vi "Apply Body Text.vi"(6 "Layer name":string, 8 "error in (no error)":errorcluster, 9 "Body test":T2 {"Body Text Spec"."Alignment" items=["left", "center", "right"]}, 10 "Path & Icon":T5, 11 "Icon in":refnum<class "Icon.lvclass">) -> (0 "error out":errorcluster, 2 "Data":T1 {"Opacity" scale=0.0..100.0}, 3 "Icon out":refnum<class "Icon.lvclass">)   [LabVIEW 2021, in "Icon.lvclass"]
doc: "Updates the Text of the Text Layer."
uses:
  <vilib>/LabVIEW Icon API/lv_icon/Classes/Icon/Icon.lvclass
  <vilib>/LabVIEW Icon API/lv_icon/Controls/Graphic.ctl
  <vilib>/LabVIEW Icon API/lv_icon/Controls/BodyText.ctl
  <vilib>/LabVIEW Icon API/lv_icon/Controls/Font.ctl
  <vilib>/LabVIEW Icon API/lv_icon/Controls/Alignment.ctl
  <vilib>/LabVIEW Icon API/lv_icon/Controls/Layer.ctl
  <vilib>/LabVIEW Icon API/lv_icon/Classes/Icon Framework/Icon Framework.lvclass
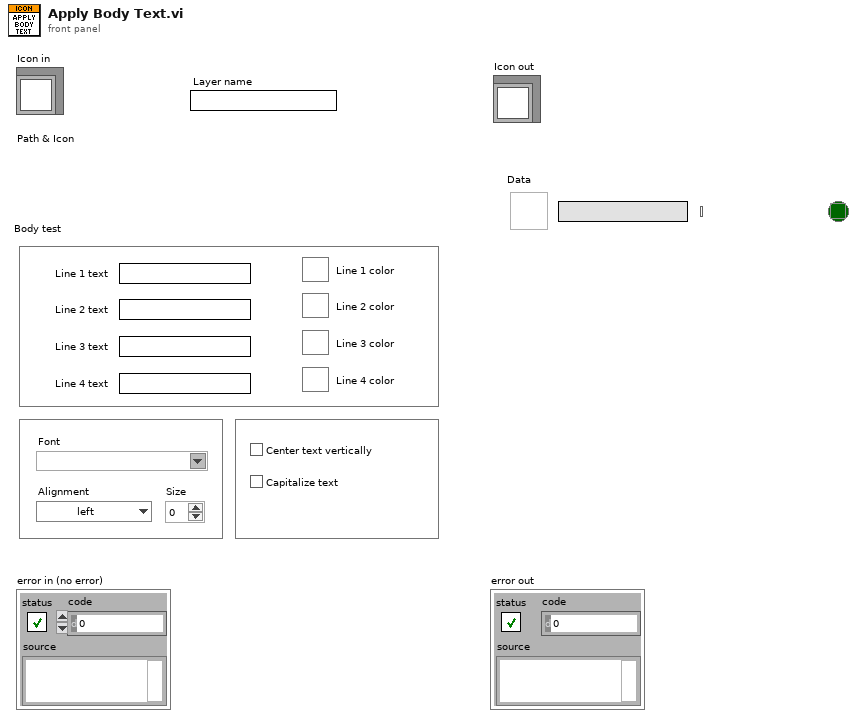
[diagram p1: front panel]
types:
  T1 = typedef "Layer.ctl" = cluster{"LayerIcon":picture, "LayerName":string, "Opacity":u8, "Visibility?":bool}
  T2 = typedef "BodyText.ctl" = cluster{"Line 1 text":string, "Line 2 text":string, "Line 3 text":string, "Line 4 text":string, "Line 1 color":u32, "Line 2 color":u32, "Line 3 color":u32, "Line 4 color":u32, "Body Text Spec":cluster{"Font":T3, "Alignment":T4, "Size":u8}, "Center text vertically":bool, "Capitalize Text":bool}
  T3 = typedef "Font.ctl" = string
  T4 = typedef "Alignment.ctl" = u16
  T5 = typedef "Graphic.ctl" = cluster{"Rectangle":cluster{"left":i16, "top":i16, "right":i16, "bottom":i16}, "Path":path, "Image":picture, "Filter":string, "FileName":string}
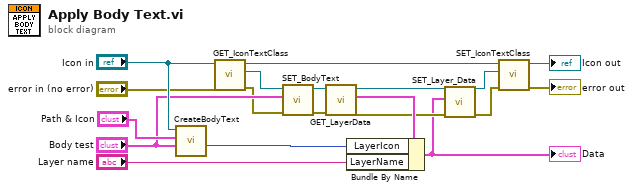
[diagram p0: block diagram]
diagram:
  n1 = call <vilib>:"CreateBodyText.vi"("Body Text"="Body test", "Path and Icon Template"="Path & Icon", "Icon.lvclass in"="Icon in") -> ("Body Text"=w17:picture)  [unwired: 1 in, 7 out]
  n2 = call-dynamic "GET_IconTextClass.vi"("error in (no error)"="error in (no error)", "Icon.lvclass in"="Icon in") -> ("error out"=w10:errorcluster, "Icon Framework.lvclass"=w11:refnum<class "Icon Framework.lvclass">, "Icon.lvclass out"=w12:refnum<class "Icon.lvclass">)  [unwired: 7 out]
  n3 = call-dynamic "SET_BodyText.vi"("error in (no error)"=w10, "Body Text"="Body test", "Icon Framework.lvclass in"=w11) -> ("error out"=w2:errorcluster, "Icon Framework.lvclass out"=w5:refnum<class "Icon Framework.lvclass">)  [unwired: 7 out]
  n4 = call-dynamic "GET_LayerData.vi"("error in (no error)"=w2, "Layer.lvclass in"=w5) -> ("error out"=w7:errorcluster, "Data"=w8:T1, "Layer.lvclass out"=w9:refnum<class "Icon Framework.lvclass">)  [unwired: 7 out]
  n5 = Bundle By Name(cluster=w8, "LayerIcon"=w17, "LayerName"="Layer name") -> (w6:T1)
  "Data" <- w6
  n6 = call-dynamic "SET_Layer_Data.vi"("error in (no error)"=w7, "Data"=w6, "Layer.lvclass in"=w9) -> ("error out"=w1:errorcluster, "Layer.lvclass out"=w4:refnum<class "Icon Framework.lvclass">)  [unwired: 1 in, 6 out]
  n7 = call-dynamic "SET_IconTextClass.vi"("error in (no error)"=w1, "Icon Framework.lvclass"=w4, "Icon.lvclass in"=w12) -> ("error out"=→"error out":errorcluster, "Icon.lvclass out"=→"Icon out":refnum<class "Icon.lvclass">)  [unwired: 7 out]
